vi "Drum Subvi April 6.vi"(0 "Yellow Line":T2={"Global Rectangle"=[342, 292, 349, 377], "Contours"=[{"ID"=enum."External", "Type"=2, "Coordinates"=[342, 376, 348, 292]}]} {"Contours"."Type" items=["No Selection", "Point", "Line", "Rectangle", "Oval", "Polygon", "Freehand Region", "Annulus", "Unused2", "Unused3", "Broken Line", "Freehand Line", "Rotated Rectangle"]}, 1 "Green Line":T2={"Global Rectangle"=[406, 309, 423, 383], "Contours"=[{"ID"=enum."External", "Type"=2, "Coordinates"=[422, 382, 406, 309]}]} {"Contours"."Type" items=["No Selection", "Point", "Line", "Rectangle", "Oval", "Polygon", "Freehand Region", "Annulus", "Unused2", "Unused3", "Broken Line", "Freehand Line", "Rotated Rectangle"]}, 3 "Red Line":T2={"Global Rectangle"=[300, 297, 320, 380], "Contours"=[{"ID"=enum."External", "Type"=2, "Coordinates"=[300, 379, 319, 297]}]} {"Contours"."Type" items=["No Selection", "Point", "Line", "Rectangle", "Oval", "Polygon", "Freehand Region", "Annulus", "Unused2", "Unused3", "Broken Line", "Freehand Line", "Rotated Rectangle"]}, 8 "Image Dst Out":T1, 12 "Blue Line":T2={"Global Rectangle"=[374, 278, 383, 377], "Contours"=[{"ID"=enum."External", "Type"=2, "Coordinates"=[382, 376, 374, 278]}]} {"Contours"."Type" items=["No Selection", "Point", "Line", "Rectangle", "Oval", "Polygon", "Freehand Region", "Annulus", "Unused2", "Unused3", "Broken Line", "Freehand Line", "Rotated Rectangle"]}, 14 "error out":errorcluster) -> (7 "Red Drum":bool, 9 "Yellow Array":bool[](array[boolean]), 13 "Foot Pedal":bool, 16 "Blue array":bool[](array[boolean]), 17 "Red Array":bool[](array[boolean]), 20 "Green Array":bool[](array[boolean]), 23 "Blue Drum 2":bool, 24 "Yellow Drum":bool, 25 "Green Drum":bool, 27 "error out 2":errorcluster)   [LabVIEW 2009]
uses:
  <vilib>/vision/Image Controls.llb/IMAQ Image.ctl
  <vilib>/Analysis/3filter.llb/Filter Passband Type.ctl
  <vilib>/Analysis/3filter.llb/Butterworth Filter (DBL).vi
  <vilib>/Analysis/NI_AALBase.lvlib
  <vilib>/vision/NI_Vision_Development_Module.lvlib
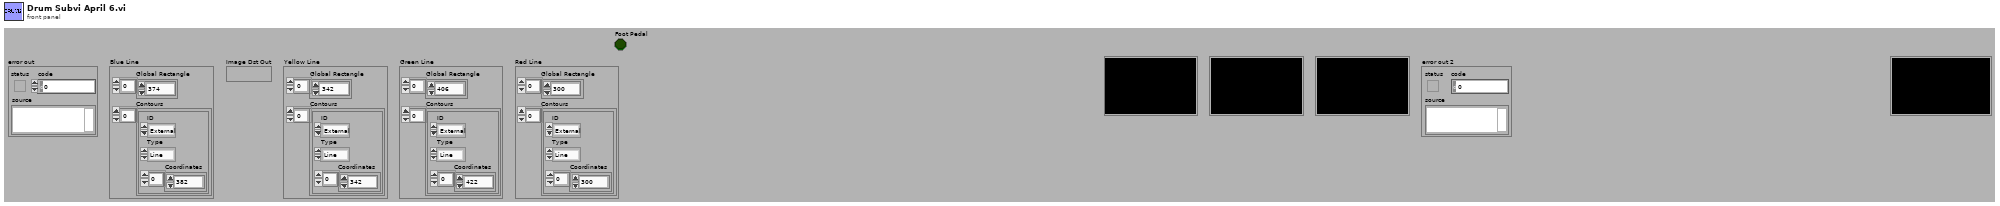
[diagram p1: front panel]
types:
  T1 = typedef "IMAQ Image.ctl" = refnum<image>
  T2 = cluster{"Global Rectangle":i32[], "Contours":cluster{"ID":enum32{"External", "Internal"}, "Type":u32, "Coordinates":i32[]}[]}
  T3 = typedef "NI_AALBase.lvlib/Filter Passband Type.ctl" = enum32{"Lowpass", "Highpass", "Bandpass", "Bandstop"}
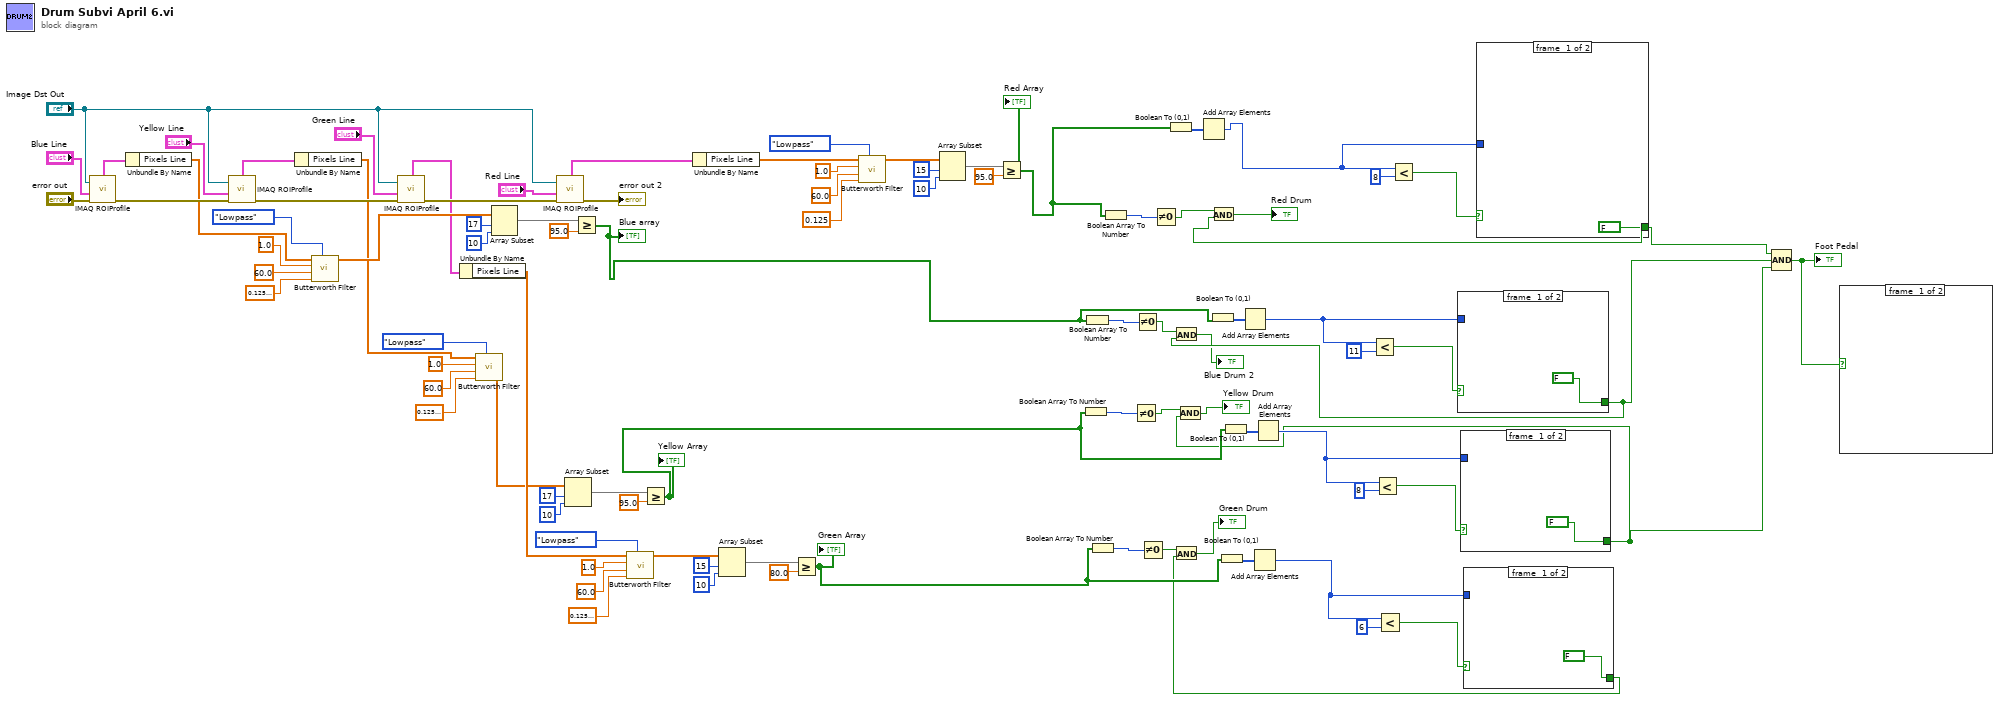
[diagram p0: block diagram]
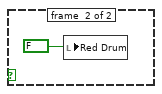
[diagram p2: hidden frame]
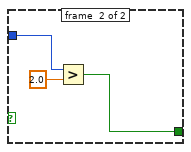
[diagram p3: hidden frame]
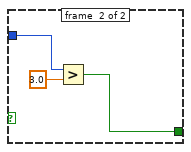
[diagram p4: hidden frame]
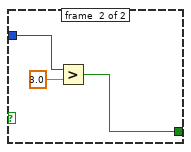
[diagram p5: hidden frame]
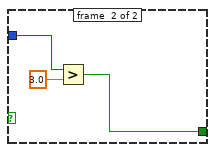
[diagram p6: hidden frame]
diagram:
  n1 = call "IMAQ ROIProfile"("error in (no error)"="error out", "ROI Descriptor"="Blue Line", "Image"="Image Dst Out") -> ("error out"=w60:errorcluster, "ROI Graph"=w61:cluster{"x0":sgl, "dx":sgl, "Pixels Line":sgl[]})  [unwired: 4 out]
  n2 = Unbundle By Name(w61) -> ("Pixels Line"=w42:sgl[])
  n3 = call "IMAQ ROIProfile"("error in (no error)"=w60, "ROI Descriptor"="Yellow Line", "Image"="Image Dst Out") -> ("error out"=w88:errorcluster, "ROI Graph"=w57:cluster{"x0":sgl, "dx":sgl, "Pixels Line":sgl[]})  [unwired: 4 out]
  n4 = Unbundle By Name(w57) -> ("Pixels Line"=w54:sgl[])
  n5 = call-poly <vilib>:"Butterworth Filter.vi"("filter type"=Filter_Passband_Type."Lowpass", "low cutoff freq: fl"=0.12500000000000006 ("low"), "high cutoff freq: fh"=60.0 ("high"), "sampling freq: fs"=1.0 ("sampling"), "X"=w42) -> ("Filtered X"=w73:dbl[])  [unwired: 3 in, 1 out]
  n6 = call "IMAQ ROIProfile"("error in (no error)"=w88, "ROI Descriptor"="Green Line", "Image"="Image Dst Out") -> ("error out"=w85:errorcluster, "ROI Graph"=w63:cluster{"x0":sgl, "dx":sgl, "Pixels Line":sgl[]})  [unwired: 4 out]
  n7 = Unbundle By Name(w63) -> ("Pixels Line"=w66:sgl[])
  n8 = call-poly <vilib>:"Butterworth Filter.vi"("filter type"=Filter_Passband_Type."Lowpass", "low cutoff freq: fl"=0.12500000000000006 ("low  2"), "high cutoff freq: fh"=60.0 ("high 2"), "sampling freq: fs"=1.0 ("sampling 2"), "X"=w54) -> ("Filtered X"=w58:dbl[])  [unwired: 3 in, 1 out]
  n9 = Array Subset(array=w73, index=17, length=10) -> (w48:dbl[])
  n10 = call "IMAQ ROIProfile"("error in (no error)"=w85, "ROI Descriptor"="Red Line", "Image"="Image Dst Out") -> ("error out"=→"error out 2":errorcluster, "ROI Graph"=w84:cluster{"x0":sgl, "dx":sgl, "Pixels Line":sgl[]})  [unwired: 4 out]
  n11 = Array Subset(array=w58, index=17, length=10) -> (w51:dbl[])
  n12 = Greater Or Equal?(x=w48, y=95.0) -> (x >= y?=w22:bool[])
  "Blue array" <- w22
  n13 = call-poly <vilib>:"Butterworth Filter.vi"("filter type"=Filter_Passband_Type."Lowpass", "low cutoff freq: fl"=0.12500000000000006 ("low  3"), "high cutoff freq: fh"=60.0 ("high 3"), "sampling freq: fs"=1.0 ("sampling 3"), "X"=w66) -> ("Filtered X"=w62:dbl[])  [unwired: 3 in, 1 out]
  n14 = Greater Or Equal?(x=w51, y=95.0) -> (x >= y?=w24:bool[])
  "Yellow Array" <- w24
  n15 = Unbundle By Name(w84) -> ("Pixels Line"=w81:sgl[])
  n16 = Array Subset(array=w62, index=15, length=10) -> (w69:dbl[])
  n17 = Greater Or Equal?(x=w69, y=80.0) -> (x >= y?=w26:bool[])
  "Green Array" <- w26
  n18 = call-poly <vilib>:"Butterworth Filter.vi"("filter type"=Filter_Passband_Type."Lowpass", "low cutoff freq: fl"=0.125 ("low  4"), "high cutoff freq: fh"=60.0 ("high 4"), "sampling freq: fs"=1.0 ("sampling 4"), "X"=w81) -> ("Filtered X"=w1:dbl[])  [unwired: 3 in, 1 out]
  n19 = Array Subset(array=w1, index=15, length=10) -> (w78:dbl[])
  n20 = Greater Or Equal?(x=w78, y=95.0) -> (x >= y?=w13:bool[])
  "Red Array" <- w13
  n21 = Boolean Array To Number(Boolean array=w24) -> (number=w37:u32)
  n22 = Boolean Array To Number(Boolean array=w22) -> (number=w38:u32)
  n23 = Boolean Array To Number(Boolean array=w26) -> (number=w36:u32)
  n24 = Boolean Array To Number(Boolean array=w13) -> (number=w14:u32)
  n25 = Not Equal To 0?(x=w37) -> (x != 0?=w11:bool)
  n26 = Not Equal To 0?(x=w38) -> (x != 0?=w9:bool)
  n27 = Not Equal To 0?(x=w36) -> (x != 0?=w10:bool)
  n28 = Not Equal To 0?(x=w14) -> (x != 0?=w12:bool)
  n29 = Boolean To (0,1)(Boolean=w13) -> (0, 1=w35:i16[])
  n30 = Add Array Elements(numeric array=w35) -> (sum=w32:i16)
  n31 = Boolean To (0,1)(Boolean=w22) -> (0, 1=w29:i16[])
  n32 = Boolean To (0,1)(Boolean=w26) -> (0, 1=w27:i16[])
  n33 = Boolean To (0,1)(Boolean=w24) -> (0, 1=w28:i16[])
  n34 = Add Array Elements(numeric array=w29) -> (sum=w21:i16)
  n35 = Add Array Elements(numeric array=w27) -> (sum=w25:i16)
  n36 = Add Array Elements(numeric array=w28) -> (sum=w23:i16)
  n37 = Less?(x=w21, y=i16 11) -> (x < y?=w31:bool)
  n38 = Less?(x=w23, y=i16 8) -> (x < y?=w20:bool)
  n39 = Less?(x=w25, y=i16 6) -> (x < y?=w17:bool)
  n40 = Less?(x=w32, y=i16 8) -> (x < y?=w33:bool)
  n41 = case shown="True" w31 {
    tunnel: w21 -> [_ w95]
    tunnel: [FALSE w94] -> w8
    frame #0 {
    }
    frame #1 {
      n42 = Greater?(x=w95, y=3.0) -> (0:w94:bool)
    }
  }
  n43 = And(x=w9, y=w8) -> (x .and. y?=→"Blue Drum 2":bool)
  n44 = case shown="True" w20 {
    tunnel: w23 -> [_ w99]
    tunnel: [FALSE w98] -> w6
    frame #0 {
    }
    frame #1 {
      n45 = Greater?(x=w99, y=3.0) -> (0:w98:bool)
    }
  }
  n46 = And(x=w11, y=w6) -> (x .and. y?=→"Yellow Drum":bool)
  n47 = case shown="True" w17 {
    tunnel: w25 -> [_ w103]
    tunnel: [FALSE w102] -> w3
    frame #0 {
    }
    frame #1 {
      n48 = Greater?(x=w103, y=2.0) -> (0:w102:bool)
    }
  }
  n49 = And(x=w10, y=w3) -> (x .and. y?=→"Green Drum":bool)
  n50 = case shown="True" w33 {
    tunnel: w32 -> [_ w106]
    tunnel: [FALSE w105] -> w16
    frame #0 {
    }
    frame #1 {
      n51 = Greater?(x=w106, y=3.0) -> (0:w105:bool)
    }
  }
  n52 = And(x=w12, y=w16) -> (x .and. y?=→"Red Drum":bool)
  n53 = Compound Arithmetic op=AND(w16, w8, w6) -> (w2:bool)
  "Foot Pedal" <- w2
  n54 = case shown="False" w2 {
    frame #0 {
    }
    frame #1 {
      n55 = local write "Red Drum"(FALSE) -> ()
    }
  }
